vi "Configure Mode.vi"(8 "error in (no error)":errorcluster, 10 "Select Mode (Normal)":u16(ring) items=["Normal", "Ballast", "Inrush", "Standby Power", "Integrator"], 11 "VISA resource name":refnum<visa-resource-name>) -> (0 "error out":errorcluster, 3 "VISA resource name out":refnum<visa-resource-name>)   [LabVIEW 2015, in "Voltech PM1000+.lvlib"]
doc: "Configures PM1000+ operation mode, set PM1000+ integration start method to \"Manual Start Method\", sets the user defined period of averaging in Low Power Standby mode, and set Default Inrush current range."
uses:
  <instrlib>/Voltech PM1000+/Voltech PM1000+.lvlib
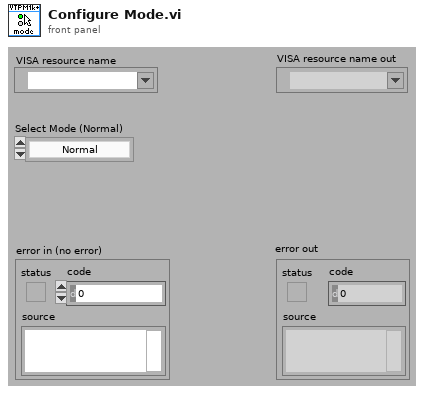
[diagram p1: front panel]
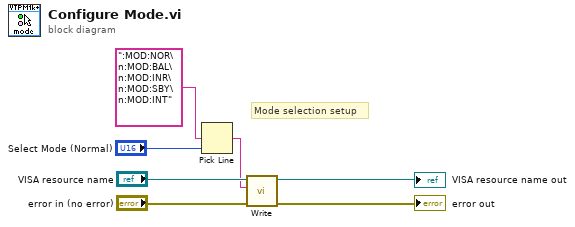
[diagram p0: block diagram]
diagram:
  # "Mode selection setup"
  n1 = Pick Line(multi-line string=":MOD:NOR\n:MOD:BAL\n:MOD:INR\n:MOD:SBY\n:MOD:INT", line index="Select Mode (Normal)") -> (output string=w3:string)  [unwired: 1 in]
  n2 = call <instrlib>:"Write.vi"("error in (no error)"="error in (no error)", "Write Buffer"=w3, "VISA resource name"="VISA resource name") -> ("error out"=→"error out":errorcluster, "VISA resource name out"=→"VISA resource name out":refnum<visa-resource-name>)  [unwired: 7 in]
